vi "Test FPGA.vi"() -> ()   [LabVIEW 2014]
uses:
  <vilib>/rvi/Emulation/niFpgaGetClockAttributes.vi
  <vilib>/rvi/Emulation/niFpgaSctlEmulationGetInTimedLoop.vi
  <vilib>/rvi/Emulation/niFpgaEmulationReportErrorSimple.vi
  <vilib>/rvi/Memory/Memory_Emulation/nirvimemoryFastEmulation.vi
  <vilib>/rvi/Memory/Memory_Emulation/nirvimemoryEmulation.vi
  <vilib>/rvi/Emulation/niFpgaEmulationIsFPGAContextNoSignature.vi
  <vilib>/rvi/DataTransferAndStorage/Container/Common/niFpgaContainerGetUniqueNameForEmu.vi
  <vilib>/rvi/Emulation/niFpgaProcessEmulError.vi
  <vilib>/rvi/errors/nirviReportUnexpectedCaseInternalError (U32).vi
  <vilib>/rvi/interface/RandomDataEmulation/niFpgaRandomDataHandleErrors.vi
  <vilib>/rvi/Emulation/niFpgaCriticalErrorInLSC.vi
  <vilib>/rvi/DataTransferAndStorage/Container/XNode/niFpgaContainer.xnode
  <vilib>/rvi/interface/RandomDataEmulation/nirviRandomDataFpgaReadWriteTemplate.vi
panel:
  in  "Stop Button":bool
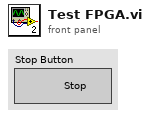
[diagram p1: front panel]
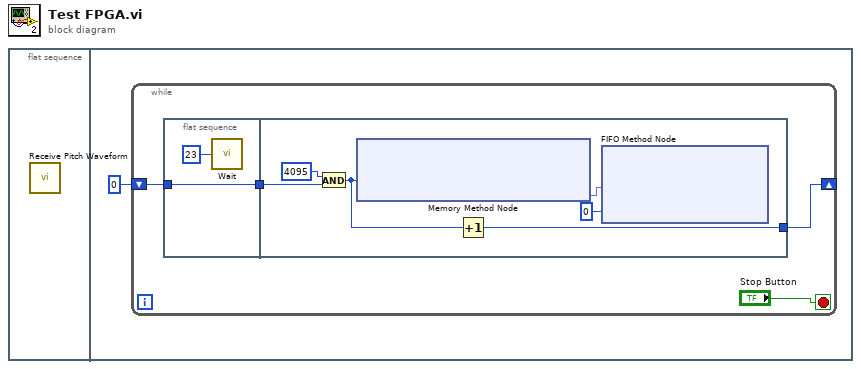
[diagram p0: block diagram]
diagram:
  n1 = flat-sequence {
    frame #0 {
      n2 = call "Receive Pitch Waveform.vi"() -> ()  [unwired: 12 in]
    }
    frame #1 {
      n3 = while {
        shift-right: [w4] -> _
        shift-left: u32 0 -> [w5]
        stop <- "Stop Button" stop-if-true
        n4 = flat-sequence {
          tunnel: w5 -> [w7]
          tunnel: [w7] -> w3
          tunnel: [w10] -> w4
          tunnel: w3 -> [w12]
          frame #0 {
            n5 = call "Wait"("Count(uSec)"=u32 23 ("Count(mSec)")) -> ()  [unwired: 1 out]
          }
          frame #1 {
            n6 = And(x=u32 4095, y=w12) -> (x .and. y?=w11:u32)
            n7 = xnode ("Memory Method Node")("Address"=w11) -> ("Data"=w9:fxp<+/-,10,2>)  [unwired: 1 in, 1 out]
            n8 = Increment(x=w11) -> (x+1=w10:u32)
            n9 = xnode ("FIFO Method Node")("Element"=w9, "Timeout"=0) -> ()  [unwired: 1 in, 2 out]
          }
        }
      }
    }
  }
